vi "编辑个人信息.vi"(9 "修改的信息":cluster{"电话":string, "邮箱":string, "备注":string}, 10 "用户名":string, 11 "数据库连接引用":T1) -> (0 "error out":errorcluster)   [LabVIEW 2013, in "数据库操作.lvclass"]
uses:
  <vilib>/addons/database/Connection.llb/Conn ObjectReference.ctl
  <vilib>/addons/database/Connection.llb/Conn Execute.vi
  <vilib>/addons/database/NI_Database_API.lvlib
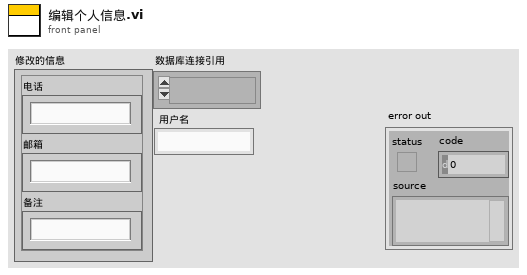
[diagram p1: front panel]
types:
  T1 = typedef "NI_Database_API.lvlib/Conn ObjectReference.ctl" = refnum<k1>
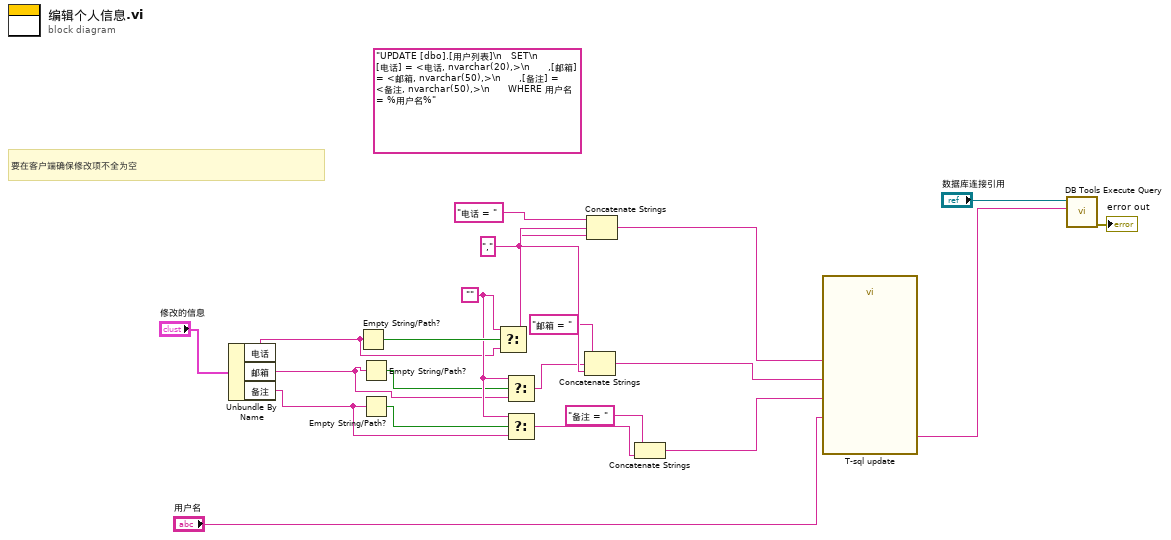
[diagram p0: block diagram]
diagram:
  w14 = ","
  w20 = ""
  (unwired) "UPDATE [dbo].[用户列表]\n   SET\n      [电话] = <电话, nvarchar(20),>\n      ,[邮箱] = <邮箱, nvarchar(50),>\n      ,[备注] = <备注, nvarchar(50),>\n      WHERE 用户名 = %用户名%"
  # "要在客户端确保修改项不全为空"
  n1 = Unbundle By Name("修改的信息") -> ("电话"=w16:string, "邮箱"=w12:string, "备注"=w10:string)
  n2 = Empty String/Path?(string/path=w16) -> (empty?=w21:bool)
  n3 = Empty String/Path?(string/path=w12) -> (empty?=w19:bool)
  n4 = Empty String/Path?(string/path=w10) -> (empty?=w18:bool)
  n5 = Select(t=w20, s=w21, f=w16) -> (s? t:f=w15:string)
  n6 = Select(t=w20, s=w19, f=w12) -> (s? t:f=w11:string)
  n7 = Select(t=w20, s=w18, f=w10) -> (s? t:f=w9:string)
  n8 = Concatenate Strings("邮箱 = ", w11, w14) -> (w6:string)
  n9 = Concatenate Strings("电话 = ", w15, w14) -> (w7:string)
  n10 = Concatenate Strings("备注 = ", w9) -> (w5:string)
  n11 = call "T-sql update"("用户名"="用户名", "电话"=w7, "邮箱"=w6, "备注"=w5) -> ("Result"=w3:string)  [unwired: 10 in, 1 out]
  n12 = call-poly <vilib>:"DB Tools Execute Query.vi"("SQL query"=w3, "connection reference"="数据库连接引用") -> ("error out"=→"error out":errorcluster)  [unwired: 6 in, 1 out]
